vi "global tas.vi"() -> ()   [LabVIEW 2015]
panel:
  in  "Root Path":path=path "D:/Data/TAS data"
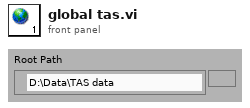
[diagram p1: front panel]
diagram:
